vi "PID Veering.vi"(6 "Error":dbl, 7 "Current Distance":dbl=15.0 format="%#_13g", 8 "error in (no error)":errorcluster, 11 "Refnum's":T1={"Gyro"="Gyro", "Mtr 1"="LeftMtr", "Mtr 2"="RightMtr"}) -> (0 "error out":errorcluster)   [LabVIEW 2016]
uses:
  <vilib>/addons/control/pid/pid.llb/PID (DBL).vi
  <vilib>/addons/control/pid/NI_PID_pid.lvlib
panel:
  out "Left":dbl
  out "Right":dbl
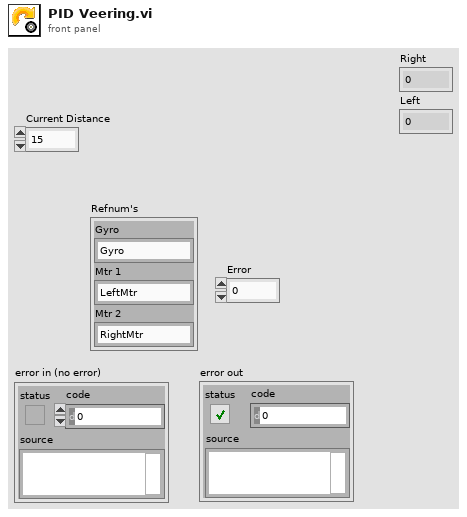
[diagram p1: front panel]
types:
  T1 = cluster{"Gyro":string, "Mtr 1":string, "Mtr 2":string}
  T2 = typedef "WPI_MotorControlDeviceRef.ctl" = cluster{"DeviceStatus":errorcluster, "Type":T3, "PWM":cluster{"PWM Channel":T4, "DeadBand":T5}, "CAN":cluster{"Device Number":u8, "SetOutput VI Ref":variant, "GetOutput VI Ref":variant, "Enable VI Ref":variant, "Disable VI Ref":variant, "Data":variant}, "Invert":bool}
  T3 = typedef "WPI_MotorControlType.ctl" = enum16{"PWM", "CAN"}
  T4 = typedef "FPGA_DIOPWMChannel.ctl" = enum8{"PWM 0", "PWM 1", "PWM 2", "PWM 3", "PWM 4", "PWM 5", "PWM 6", "PWM 7", "PWM 8", "PWM 9", "PWM MXP 0", "PWM MXP 1", "PWM MXP 2", "PWM MXP 3", "PWM MXP 4", "PWM MXP 5", "PWM MXP 6", "PWM MXP 7", "PWM MXP 8", "PWM MXP 9", "Invalid"}
  T5 = typedef "WPI_PWMDeadband.ctl" = cluster{"Name":string, "maxPositivePwm":i32, "minPositivePwm":i32, "centerPwm":i32, "maxNegativePwm":i32, "minNegativePwm":i32, "angularRange":u16}
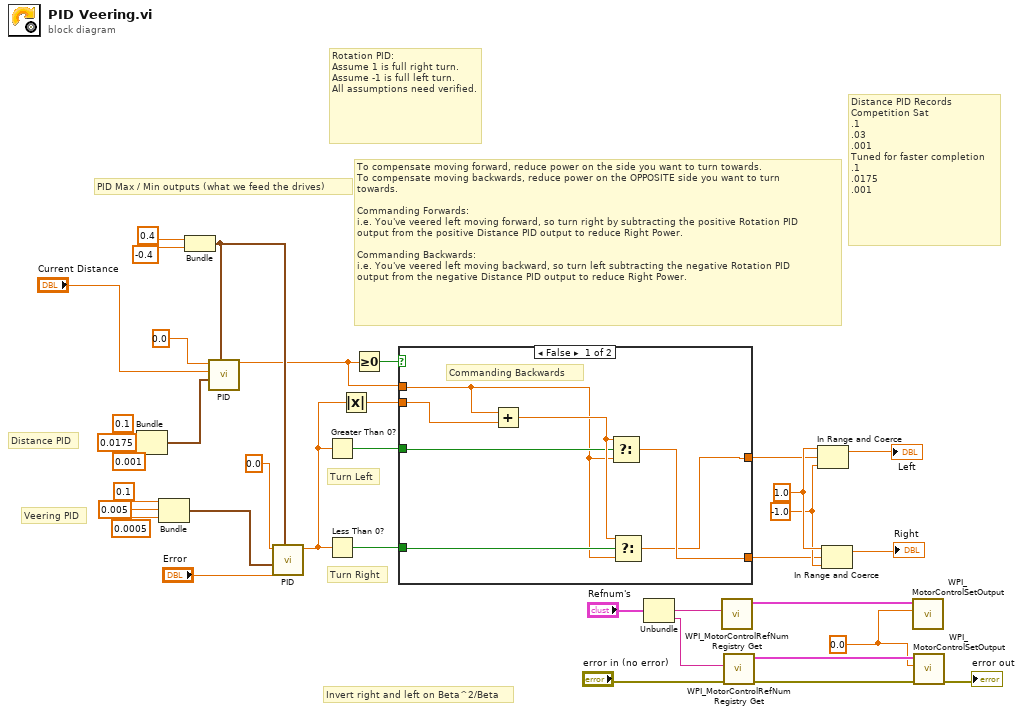
[diagram p0: block diagram]
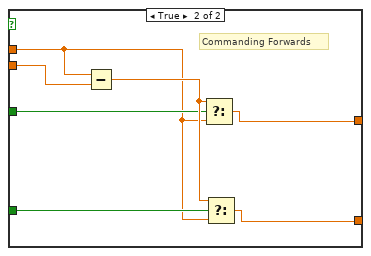
[diagram p2: hidden frame]
diagram:
  w1 = 0.0 ("Output")
  w21 = -1.0
  w22 = 1.0
  # "Veering PID"
  # "Distance PID"
  # "Distance PID Records\nCompetition Sat\n.1\n.03\n.001\nTuned for faster completion\n.1\n.0175\n.001"
  # "Invert right and left on Beta^2/Beta"
  # "Turn Right"
  # "Turn Left"
  # "To compensate moving forward, reduce power on the side you want to turn towards.\nTo compensate moving backwards, reduce power on the OPPOSITE side you want to turn\ntowards.\n\nCommanding Forwards:\ni.e. You've veered left moving forward, so turn right by subtracting the positive Rotation PID\noutput from the positive Distance PID output to reduce Right Power.\n\nCommanding Backwards:\ni.e. You've veered left moving backward, so turn left subtracting the negative Rotation PID \noutput from the negative Distance PID output to reduce Right Power."
  # "PID Max / Min outputs (what we feed the drives)"
  # "Rotation PID:\nAssume 1 is full right turn.\nAssume -1 is full left turn.\nAll assumptions need verified."
  n1 = Bundle(0.1, 0.0175, 0.001) -> (w29:cluster{dbl, dbl, dbl})  [unwired: 1 in]
  n2 = Bundle(0.1, 0.005, 0.0005) -> (w25:cluster{dbl, dbl, dbl})  [unwired: 1 in]
  n3 = Bundle(0.4, -0.4) -> (w24:cluster{dbl, dbl})  [unwired: 1 in]
  n4 = call-poly <vilib>:"PID.vi"("output range"=w24, "PID gains"=w29, "process variable"="Current Distance", "setpoint"=0.0) -> ("output"=w20:dbl)  [unwired: 6 in, 1 out]
  n5 = call-poly <vilib>:"PID.vi"("output range"=w24, "PID gains"=w25, "process variable"="Error", "setpoint"=0.0) -> ("output"=w14:dbl)  [unwired: 6 in, 1 out]
  n6 = Greater Than 0?(x=w14) -> (x > 0?=w16:bool)
  n7 = Less Than 0?(x=w14) -> (x < 0?=w15:bool)
  n8 = Absolute Value(x=w14) -> (abs(x)=w19:dbl)
  n9 = Greater Or Equal To 0?(x=w20) -> (x >= 0?=w23:bool)
  n10 = case shown="False" w23 {
    tunnel: w19 -> [w40 w50]
    tunnel: w20 -> [w37 w44]
    tunnel: [w39 w48] -> w18
    tunnel: [w38 w47] -> w17
    tunnel: w16 -> [w42 w46]
    tunnel: w15 -> [w41 w45]
    frame False {
      # "Commanding Backwards"
      n11 = Add(x=w37, y=w40) -> (x+y=w43:dbl)
      n12 = Select(t=w43, s=w42, f=w37) -> (s? t:f=w39:dbl)
      n13 = Select(t=w43, s=w41, f=w37) -> (s? t:f=w38:dbl)
    }
    frame True {
      # "Commanding Forwards"
      n14 = Subtract(x=w44, y=w50) -> (x-y=w49:dbl)
      n15 = Select(t=w49, s=w46, f=w44) -> (s? t:f=w47:dbl)
      n16 = Select(t=w49, s=w45, f=w44) -> (s? t:f=w48:dbl)
    }
  }
  n17 = Unbundle("Refnum's") -> ("Mtr 1"=w36:string, "Mtr 2"=w35:string)  [unwired: 1 out]
  n18 = call <vilib>:"WPI_MotorControlRefNum Registry Get.vi"("refnum name"=w36) -> ("MotorControlDevRef"=w9:T2)  [unwired: 9 in, 1 out]
  n19 = call <vilib>:"WPI_MotorControlRefNum Registry Get.vi"("error in (no error)"="error in (no error)", "refnum name"=w35) -> ("error out"=w4:errorcluster, "MotorControlDevRef"=w10:T2)  [unwired: 8 in]
  n20 = In Range and Coerce(upper limit=w22, x=w17, lower limit=w21) -> (coerced(x)=→"Left":dbl)  [unwired: 1 out]
  n21 = In Range and Coerce(upper limit=w22, x=w18, lower limit=w21) -> (coerced(x)=→"Right":dbl)  [unwired: 1 out]
  n22 = call <vilib>:"WPI_MotorControlSetOutput.vi"("Output"=w1, "MotorControlDevRef"=w9) -> ()  [unwired: 7 in, 3 out]
  n23 = call <vilib>:"WPI_MotorControlSetOutput.vi"("error in (no error)"=w4, "Output"=w1, "MotorControlDevRef"=w10) -> ("error out"=→"error out":errorcluster)  [unwired: 6 in, 2 out]
